vi "Sequencer Main.vi"() -> ()   [LabVIEW 2018] (continued)
              n953 = local read "Barcode"() -> (w1433:string)
              n954 = String Length(string=w1433) -> (length=w1436:i32)
              n955 = Greater?(x=w1436, y=5) -> (0:w1434:bool)
              n956 = case shown="True" w1434 {
                tunnel: w1433 -> [_ w1445]
                tunnel: ["Barcode Err!" w1444] -> w1432
                frame False {
                  n957 = in-place {
                    n958 = global write "Global Variable.vi" "System Status"(T1."Idle" ("System Status")) -> ()
                  }
                  n959 = global write "Global Variable.vi" "Reset BARCODE"(FALSE ("Reset BARCODE")) -> ()
                  n960 = One Button Dialog(message="! - Please Read BARCODE First") -> ()  [unwired: 1 in, 1 out]
                }
                frame True {
                  w1443 = "----------------------------------"
                  w1442 = "\r\n"
                  w1446 = ", "
                  n961 = in-place {
                    n962 = global write "Global Variable.vi" "System Status"(T1."Run Sequencer" ("System Status")) -> ()
                  }
                  n963 = local read "Under Test BOARD"() -> (w1448:string)
                  n964 = local read "Date Time"() -> (w1441:string)
                  n965 = local read "Config"() -> (w1447:string)
                  n966 = global write "Global Variable.vi" "Reset BARCODE"(TRUE ("Reset BARCODE")) -> ()
                  n967 = property on="Run Test" class="Bool"("DisabledEnum"=T18."Disabled and Grayed Out" ("Disabled")) -> ()  [unwired: 2 in, 2 out]
                  n968 = Concatenate Strings(w1448, w1446, w1447, w1446, w1445, w1442, w1443, w1442, w1441, w1442, w1443, w1443, w1442, w1442) -> (w1444:string)
                }
              }
              n969 = local write "LogMsg"(w1432) -> ()
            }
          }
        }
        frame "Run Sequencer" {
          n970 = global read "Sequencer Array.vi" "SEQUENCER Array"() -> (w1452:T16[])
          n971 = Array Size(array=w1452) -> (size(s)=w1457:i32)
          n972 = global write "Global Variable.vi" "Steps Nmb"(w1457) -> ()
          n973 = Greater Than 0?(x=w1457) -> (x > 0?=w1458:bool)
          n974 = case shown="True" w1458 {
            tunnel: w1453 -> [w1461 w1484]
            tunnel: w1456 -> [w1460 w1483]
            tunnel: w1452 -> [_ w1482]
            tunnel: w1453 -> [_ w1475]
            tunnel: w1455 -> [_ w1470]
            tunnel: w1454 -> [_ w1469]
            frame False {
              # "Empty TEST Sequencer"
              n975 = Flush Queue(queue=w1461, error in (no error)=w1460) -> ()  [unwired: 3 out]
              n976 = One Button Dialog(message="Please Load SEQUENCER File") -> ()  [unwired: 1 in, 1 out]
              n977 = global write "Global Variable.vi" "System Status"(T1."Idle" ("System Status")) -> ()
            }
            frame True {
              # "Sys Dig In/Out"
              n978 = Dequeue Element(queue=w1484, error in (no error)=w1483) -> (element=w1466:i32, error out=w1472:errorcluster)  [unwired: 1 in, 2 out]
              n979 = Index Array(array=w1482, index=w1466) -> (element=w1480:T16)
              n980 = global write "Global Variable.vi" "Current Step Nmb"(w1466) -> ()
              n981 = property on="Test Sequencer" class="MCListbox (strict)"("Value"=w1466) -> ()  [unwired: 2 in, 2 out]
              n982 = Unbundle By Name(w1480) -> ("Run/Skip"=w1479:bool, "Step ID"=w1481:u16)
              n983 = flat-sequence {
                tunnel: w1481 -> [w1493]
                tunnel: w1480 -> [w1491]
                tunnel: w1479 -> [w1492]
                tunnel: [w1491] -> w1478
                tunnel: [w1486] -> w1476
                tunnel: w1475 -> [w1486]
                tunnel: w1472 -> [w1485]
                tunnel: [w1490] -> w1473
                tunnel: w1470 -> [w1489]
                tunnel: w1469 -> [w1488]
                tunnel: [w1487] -> w1468
                tunnel: [w1485] -> w1467
                tunnel: w1478 -> [w5997]
                tunnel: [w5996] -> w1477
                tunnel: w1476 -> [w5990]
                tunnel: [w5993] -> w1474
                tunnel: w1473 -> [w5983]
                tunnel: [w5987] -> w1471
                tunnel: w1468 -> [w5991]
                tunnel: w1467 -> [w5992]
                tunnel: [w5983] -> w1465
                tunnel: [w5985] -> w1464
                tunnel: [w5984] -> w1463
                tunnel: w1477 -> [w6131]
                tunnel: w1474 -> [w6124]
                tunnel: w1471 -> [w6129]
                tunnel: w1465 -> [w6128]
                tunnel: w1464 -> [w6123]
                tunnel: w1463 -> [w6130]
                frame #0 {
                  # "Sequencer Array Element"
                  # "Test STEPS Processor"
                  n984 = case shown="True" w1492 {
                    tunnel: w1493 -> [_ w1500]
                    tunnel: w1491 -> [_ w1499]
                    tunnel: [enum16{"Idle", "PASS", "FALSE"}."Idle" ("Step Test Result") w1498] -> w1490
                    tunnel: w1489 -> [_ w1497]
                    tunnel: w1488 -> [_ w1496]
                    tunnel: [_ w1495] -> w1487
                    frame False {
                      # "Step TEST Result"
                    }
                    frame True {
                      # "Run \\ Skip"
                      n985 = case shown="51" w1500 {
                        tunnel: w1499 -> [_ w1505 w1506 w1521 w1647 w1763 w1836 w1998 w2009 w2046 w2131 w2328 w2470 w2603 w2713 w3078 w3442 w3693 w3833 w3925 w4012 w4178 w4330 w4472 w4601 w4710 w5916 w5941]
                        tunnel: [enum16{"Idle", "PASS", "FALSE"}."Idle" ("Step Test Result") enum16{"Idle", "PASS", "FALSE"}."Idle" ("Step Test Result") enum16{"Idle", "PASS", "FALSE"}."Idle" ("Step Test Result") w1509 enum16{"Idle", "PASS", "FALSE"}."Idle" ("Step Test Result") enum16{"Idle", "PASS", "FALSE"}."Idle" ("Step Test Result") w1824 enum16{"Idle", "PASS", "FALSE"}."Idle" ("Step Test Result") enum16{"Idle", "PASS", "FALSE"}."Idle" ("Step Test Result") w2048 w2123 w2327 w2469 w2602 w2710 w3079 w3443 w3694 w3818 w3916 w3991 w4161 w4311 w4466 w4592 w4707 w5907 enum16{"Idle", "PASS", "FALSE"}."PASS" ("Step Test Result")] -> w1498
                        tunnel: w1497 -> [_ _ _ w1515 w1640 w1756 w1829 _ _ _ _ _ _ _ _ _ _ _ _ _ _ _ _ _ _ _ _ w5934]
                        tunnel: w1496 -> [_ _ _ w1514 w1639 w1755 w1828 _ _ _ _ _ _ _ _ _ _ _ _ _ _ _ _ _ _ _ _ w5933]
                        tunnel: [_ _ _ _ _ _ _ _ _ w2045 w2124 w2324 w2466 w2599 w2686 w3071 w3429 w3680 w3817 _ w3990 w4160 w4310 w4465 "SetAWG Gen" ("format string") w4683 w5904 _] -> w1495
                        frame 0, Default {
                          # "Step TEST Result"
                          n986 = One Button Dialog(message="Wrong Step ID!") -> ()  [unwired: 1 in, 1 out]
                        }
                        frame 1 {
                          # "Step TEST Result"
                          # "Label Case"
                          # "Step ID Processing"
                          n987 = Unbundle By Name(w1505) -> ("Step Description"=w1504:string)
                          n988 = local write "Message"(w1504) -> ()
                        }
                        frame 5 {
                          # "Step TEST Result"
                          # "Barcode Case"
                          # "Barcode Operation"
                          n989 = Unbundle By Name(w1506) -> ("Step Description"=w1508:string)
                          n990 = local write "Message"(w1508) -> ()
                        }
                        frame 10 {
                          # "GPIO Case"
                          # "SPI SET Relay"
                          n991 = Unbundle By Name(w1521) -> ("Parameters"=w1520:string, "Step Description"=w1512:string)
                          n992 = global write "Global Variable.vi" "GPIO Mode LUT"(bool[] [FALSE, FALSE, FALSE, FALSE] ("GPIO Mode LUT")) -> ()
                          n993 = call <vilib>:"Acquire Semaphore.vi"("error in (no error)"=w1515, "semaphore"=w1514) -> ("error out"=w1519:errorcluster, "semaphore out"=w1517:T13)  [unwired: 3 in, 1 out]
                          n994 = property on="Msg Str" class="Str"("Value"=w1512) -> ()  [unwired: 2 in, 2 out]
                          n995 = property on="Tab Control Msg" class="TabCtl (strict)"("Value"=T21."Settings" ("Tab Control Msg")) -> (error out=w1513:errorcluster)  [unwired: 2 in, 1 out]
                          n996 = case shown="No Error" w1519 {
                            selector: w1519 -> [w1524 w1634]
                            tunnel: w1520 -> [w1525 _]
                            tunnel: [w1524 w1634] -> w1518
                            tunnel: w1517 -> [w1523 w1633]
                            tunnel: [w1523 w1633] -> w1516
                            tunnel: w1513 -> [_ _]
                            tunnel: [w1522 enum16{"Idle", "PASS", "FALSE"}."Idle" ("Step Test Result")] -> w1509
                            frame No Error {
                              n997 = while {
                                shift-right: [w1530] -> _
                                shift-left: w1525 -> [w1531]
                                tunnel: [w1526] -> w1522
                                stop <- w1529 stop-if-true
                                # "Get Array of Parametrs"
                                n998 = Match Pattern(string=w1531, regular expression=";") -> (before substring=w1527:string, after substring=w1530:string, offset past match=w1528:i32)  [unwired: 1 in, 1 out]
                                n999 = Less Or Equal To 0?(x=w1528) -> (x <= 0?=w1529:bool)
                                n1000 = in-place {
                                in-place-border: w1527 -> [w1567]
                                in-place-border: [w1544] -> w1526
                                # "If True Using\nExtra Settings\n  -nCS <0-4>\n  -ClockRate"
                                # "nCS"
                                # "Addr"
                                n1001 = global read "Global Variable.vi" "GPIO Mode LUT"() -> (w1560:bool[])
                                n1002 = while {
                                shift-right: [w1629] -> _
                                shift-left: w1567 -> [w1630]
                                tunnel: [w1626] -> w1576 mode=indexing
                                stop <- w1628 stop-if-true
                                # "Get Array of Parametrs"
                                n1003 = Match Pattern(string=w1630, regular expression=">") -> (before substring=w1626:string, after substring=w1629:string, offset past match=w1627:i32)  [unwired: 1 in, 1 out]
                                n1004 = Less Than 0?(x=w1627) -> (x < 0?=w1628:bool)
                                }
                                n1005 = Index Array(array=w1576, index #1=0 ("index"), index #2=1 ("index"), index #3=2 ("index")) -> (element #1=w1577:string, element #2=w1578:string, element #3=w1561:string)
                                n1006 = Match Pattern(string=w1561, regular expression="d:") -> (after substring=w1550:string, offset past match=w1566:i32)  [unwired: 1 in, 2 out]
                                n1007 = Match Pattern(string=w1561, regular expression="b:") -> (after substring=w1549:string, offset past match=w1579:i32)  [unwired: 1 in, 2 out]
                                n1008 = Match Pattern(string=w1561, regular expression="s:") -> (after substring=w1547:string, offset past match=w1565:i32)  [unwired: 1 in, 2 out]
                                n1009 = Match Pattern(string=w1561, regular expression="r:") -> (after substring=w1546:string, offset past match=w1562:i32)  [unwired: 1 in, 2 out]
                                n1010 = Greater Than 0?(x=w1566) -> (x > 0?=w1558:bool)
                                n1011 = Greater Than 0?(x=w1562) -> (x > 0?=w1554:bool)
                                n1012 = Greater Than 0?(x=w1579) -> (x > 0?=w1556:bool)
                                n1013 = Greater Than 0?(x=w1565) -> (x > 0?=w1555:bool)
                                n1014 = Replace Array Subset(array=w1560, new element #1=w1558, index #1=0 ("index"), new element #2=w1556, index #2=1 ("index"), new element #3=w1555, index #3=2 ("index"), new element #4=w1554, index #4=3 ("index")) -> (w1548:bool[])
                                n1015 = Boolean Array To Number(Boolean array=w1548) -> (number=w1551:u32)
                                n1016 = case shown="4" w1551 {
                                tunnel: [T24."Set Decimal" ("Mode") T24."Set Decimal" ("Mode") T24."Set Binary" ("Mode") T24."Set Channels" ("Mode") T24."Reset Channels" ("Mode")] -> w1541
                                tunnel: w1550 -> [_ w1610 _ _ _]
                                tunnel: [0 w1609 0 0 0] -> w1536
                                tunnel: [bool[] [FALSE, FALSE, FALSE, FALSE, FALSE, FALSE, FALSE, FALSE, FALSE, FALSE] ("Relays (1-10)") bool[] [FALSE, FALSE, FALSE, FALSE, FALSE, FALSE, FALSE, FALSE, FALSE, FALSE] ("Relays (1-10)") w1614 w1619 w1624] -> w1535
                                tunnel: w1549 -> [_ _ w1612 _ _]
                                tunnel: w1547 -> [_ _ _ w1617 _]
                                tunnel: w1546 -> [_ _ _ _ w1622]
                                frame 0, Default {
                                # "Reset All"
                                n1017 = One Button Dialog(message="Sequencer File Err!") -> ()  [unwired: 1 in, 1 out]
                                }
                                frame 1 {
                                # "Decimale Case"
                                n1018 = Decimal String To Number(string=w1610) -> (number=w1609:i32)  [unwired: 2 in, 1 out]
                                }
                                frame 2 {
                                # "Set Binary Cnannels"
                                n1019 = call "StrBin_To_ArrayBool.vi"("StrBin"=w1612) -> ("Out"=w1615:bool[])  [unwired: 9 in, 1 out]
                                n1020 = Reverse 1D Array(array=w1615) -> (reversed array=w1614:bool[])
                                }
                                frame 4 {
                                # "Set Channels"
                                n1021 = call "StrBin_To_ArrayBool.vi"("StrBin"=w1617) -> ("Out"=w1620:bool[])  [unwired: 9 in, 1 out]
                                n1022 = Reverse 1D Array(array=w1620) -> (reversed array=w1619:bool[])
                                }
                                frame 8 {
                                # "Rest Channels"
                                n1023 = call "StrBin_To_ArrayBool.vi"("StrBin"=w1622) -> ("Out"=w1625:bool[])  [unwired: 9 in, 1 out]
                                n1024 = Reverse 1D Array(array=w1625) -> (reversed array=w1624:bool[])
                                }
                                }
                                n1025 = global write "Global Variable.vi" "GPIO Mode LUT"(w1548) -> ()
                                n1026 = Decimal String To Number(string=w1577) -> (number=w1538:i32)  [unwired: 2 in, 1 out]
                                n1027 = Decimal String To Number(string=w1578) -> (number=w1537:i32)  [unwired: 2 in, 1 out]
                                n1028 = global read "Global Variable.vi" "FTDI SPI Handle"() -> (w1542:u32)
                                n1029 = call "FTDI SPI GPIO Set.vi"("nCS"=w1538, "Relays (1-10)"=w1535, "Mode"=w1541, "Use Extra"=TRUE, "Channel Decimal"=w1536, "Addr"=w1537, "Handler In"=w1542) -> ("error out"=w1543:errorcluster, "LATCH Reg"=w1539:u16, "OK"=w1534:bool)  [unwired: 1 in, 1 out]
                                n1030 = Number To Boolean Array(number=w1539) -> (Boolean array=w1545:bool[])
                                n1031 = global write "Global Variable.vi" "Sys ERR"(w1534) -> ()
                                n1032 = case shown="4" w1537 {
                                tunnel: w1545 -> [_ w1582 w1585 w1588 w1591 w1594 w1597 w1600]
                                frame -1, Default {
                                }
                                frame 0 {
                                n1033 = local read "Switch Relay Modules"() -> (w1584:T5)
                                n1034 = Bundle By Name(cluster=w1584, "SW 0"=w1582) -> (w1583:T5)
                                n1035 = local write "Switch Relay Modules"(w1583) -> ()
                                }
                                frame 1 {
                                n1036 = local read "Switch Relay Modules"() -> (w1587:T5)
                                n1037 = Bundle By Name(cluster=w1587, "SW 1"=w1585) -> (w1586:T5)
                                n1038 = local write "Switch Relay Modules"(w1586) -> ()
                                }
                                frame 2 {
                                n1039 = local read "Switch Relay Modules"() -> (w1590:T5)
                                n1040 = Bundle By Name(cluster=w1590, "SW 2"=w1588) -> (w1589:T5)
                                n1041 = local write "Switch Relay Modules"(w1589) -> ()
                                }
                                frame 3 {
                                n1042 = local read "Switch Relay Modules"() -> (w1593:T5)
                                n1043 = Bundle By Name(cluster=w1593, "SW 3"=w1591) -> (w1592:T5)
                                n1044 = local write "Switch Relay Modules"(w1592) -> ()
                                }
                                frame 4 {
                                n1045 = local read "Switch Relay Modules"() -> (w1596:T5)
                                n1046 = Bundle By Name(cluster=w1596, "SW 4"=w1594) -> (w1595:T5)
                                n1047 = local write "Switch Relay Modules"(w1595) -> ()
                                }
                                frame 5 {
                                n1048 = local read "Switch Relay Modules"() -> (w1599:T5)
                                n1049 = Bundle By Name(cluster=w1599, "SW 5"=w1597) -> (w1598:T5)
                                n1050 = local write "Switch Relay Modules"(w1598) -> ()
                                }
                                frame 6 {
                                n1051 = local read "Switch Relay Modules"() -> (w1602:T5)
                                n1052 = Bundle By Name(cluster=w1602, "SW 6"=w1600) -> (w1601:T5)
                                n1053 = local write "Switch Relay Modules"(w1601) -> ()
                                }
                                }
                                n1054 = global read "Global Variable.vi" "Array Errors"() -> (w1574:errorcluster[])
                                n1055 = case shown="True" w1534 {
                                tunnel: [enum16{"Idle", "PASS", "FALSE"}."Idle" ("Step Test Result") enum16{"Idle", "PASS", "FALSE"}."Idle" ("Step Test Result")] -> w1544
                                frame False {
                                # "Step TEST Result"
                                }
                                frame True {
                                # "Step TEST Result"
                                }
                                }
                                n1056 = Replace Array Subset(array=w1574, new element=w1543, index=10) -> (w1575:errorcluster[])
                                n1057 = global write "Global Variable.vi" "Array Errors"(w1575) -> ()
                                n1058 = Wait (ms)(milliseconds to wait=u32 50) -> ()  [unwired: 1 out]
                                }
                              }
                            }
                            frame Error {
                              # "Step TEST Result"
                            }
                          }
                          n1059 = call <vilib>:"Release Semaphore.vi"("error in (no error)"=w1518, "semaphore"=w1516) -> ()  [unwired: 4 in, 2 out]
                        }
                        frame 11 {
                          # "GPIO SYS Case"
                          # "Step TEST Result"
                          # "SPI SET DIGOUT SYS"
                          n1060 = Unbundle By Name(w1647) -> ("Parameters"=w1645:string, "Step Description"=w1637:string)
                          n1061 = global write "Global Variable.vi" "GPIO Mode LUT"(bool[] [FALSE, FALSE, FALSE, FALSE] ("GPIO Mode LUT")) -> ()
                          n1062 = property on="Tab Control Msg" class="TabCtl (strict)"("Value"=T21."Msg" ("Tab Control Msg")) -> (error out=w1638:errorcluster)  [unwired: 2 in, 1 out]
                          n1063 = call <vilib>:"Acquire Semaphore.vi"("error in (no error)"=w1640, "semaphore"=w1639) -> ("error out"=w1644:errorcluster, "semaphore out"=w1642:T13)  [unwired: 3 in, 1 out]
                          n1064 = property on="Msg Str" class="Str"("Value"=w1637) -> ()  [unwired: 2 in, 2 out]
                          n1065 = case shown="No Error" w1644 {
                            selector: w1644 -> [w1649 w1750]
                            tunnel: w1645 -> [w1650 _]
                            tunnel: [w1649 w1750] -> w1643
                            tunnel: w1642 -> [w1648 w1749]
                            tunnel: [w1648 w1749] -> w1641
                            tunnel: w1638 -> [_ _]
                            frame No Error {
                              n1066 = while {
                                shift-right: [w1654] -> _
                                shift-left: w1650 -> [w1655]
                                stop <- w1653 stop-if-true
                                # "Get Array of Parametrs"
                                n1067 = Match Pattern(string=w1655, regular expression=";") -> (before substring=w1651:string, after substring=w1654:string, offset past match=w1652:i32)  [unwired: 1 in, 1 out]
                                n1068 = Less Or Equal To 0?(x=w1652) -> (x <= 0?=w1653:bool)
                                n1069 = in-place {
                                in-place-border: w1651 -> [w1686]
                                # "If True Using\nExtra Settings\n  -nCS <0-4>\n  -ClockRate"
                                # "nCS"
                                # "Addr"
                                n1070 = global read "Global Variable.vi" "GPIO Mode LUT"() -> (w1679:bool[])
                                n1071 = while {
                                shift-right: [w1746] -> _
                                shift-left: w1686 -> [w1747]
                                tunnel: [w1743] -> w1695 mode=indexing
                                stop <- w1745 stop-if-true
                                # "Get Array of Parametrs"
                                n1072 = Match Pattern(string=w1747, regular expression=">") -> (before substring=w1743:string, after substring=w1746:string, offset past match=w1744:i32)  [unwired: 1 in, 1 out]
                                n1073 = Less Than 0?(x=w1744) -> (x < 0?=w1745:bool)
                                }
                                n1074 = Index Array(array=w1695, index #1=0 ("index"), index #2=1 ("index"), index #3=2 ("index")) -> (element #1=w1696:string, element #2=w1697:string, element #3=w1680:string)
                                n1075 = Match Pattern(string=w1680, regular expression="d:") -> (after substring=w1669:string, offset past match=w1685:i32)  [unwired: 1 in, 2 out]
                                n1076 = Match Pattern(string=w1680, regular expression="b:") -> (after substring=w1668:string, offset past match=w1698:i32)  [unwired: 1 in, 2 out]
                                n1077 = Match Pattern(string=w1680, regular expression="s:") -> (after substring=w1666:string, offset past match=w1684:i32)  [unwired: 1 in, 2 out]
                                n1078 = Match Pattern(string=w1680, regular expression="r:") -> (after substring=w1665:string, offset past match=w1681:i32)  [unwired: 1 in, 2 out]
                                n1079 = Greater Than 0?(x=w1685) -> (x > 0?=w1677:bool)
                                n1080 = Greater Than 0?(x=w1681) -> (x > 0?=w1673:bool)
                                n1081 = Greater Than 0?(x=w1698) -> (x > 0?=w1675:bool)
                                n1082 = Greater Than 0?(x=w1684) -> (x > 0?=w1674:bool)
                                n1083 = Replace Array Subset(array=w1679, new element #1=w1677, index #1=0 ("index"), new element #2=w1675, index #2=1 ("index"), new element #3=w1674, index #3=2 ("index"), new element #4=w1673, index #4=3 ("index")) -> (w1667:bool[])
                                n1084 = Boolean Array To Number(Boolean array=w1667) -> (number=w1670:u32)
                                n1085 = case shown="0, Default" w1670 {
                                tunnel: [T23."Set Decimal" ("Mode") T23."Set Decimal" ("Mode") T23."Set Binary" ("Mode") T23."Set Channels" ("Mode") T23."Reset Channels" ("Mode")] -> _
                                tunnel: w1669 -> [_ w1726 _ _ _]
                                tunnel: [0 w1725 0 0 0] -> _
                                tunnel: [bool[] [FALSE, FALSE, FALSE, FALSE, FALSE, FALSE, FALSE, FALSE, FALSE, FALSE] ("Relays (1-10)") bool[] [FALSE, FALSE, FALSE, FALSE, FALSE, FALSE, FALSE, FALSE, FALSE, FALSE] ("Relays (1-10)") w1730 w1735 w1741] -> w1657
                                tunnel: w1668 -> [_ _ w1728 _ _]
                                tunnel: w1666 -> [_ _ _ w1733 _]
                                tunnel: w1665 -> [_ _ _ _ w1739]
                                frame 0, Default {
                                n1086 = One Button Dialog(message="Sequencer File Err!") -> ()  [unwired: 1 in, 1 out]
                                }
                                frame 1 {
                                # "Decimale Case"
                                n1087 = Decimal String To Number(string=w1726) -> (number=w1725:i32)  [unwired: 2 in, 1 out]
                                }
                                frame 2 {
                                # "Set Binary Cnannels"
                                n1088 = call "StrBin_To_ArrayBool.vi"("StrBin"=w1728) -> ("Out"=w1732:bool[])  [unwired: 9 in, 1 out]
                                n1089 = Reverse 1D Array(array=w1732) -> (reversed array=w1730:bool[])
                                }
                                frame 4 {
                                # "Set Channels"
                                n1090 = call "StrBin_To_ArrayBool.vi"("StrBin"=w1733) -> ("Out"=w1737:bool[])  [unwired: 9 in, 1 out]
                                n1091 = Reverse 1D Array(array=w1737) -> (reversed array=w1735:bool[])
                                }
                                frame 8 {
                                # "Rest Channels"
                                n1092 = call "StrBin_To_ArrayBool.vi"("StrBin"=w1739) -> ("Out"=w1742:bool[])  [unwired: 9 in, 1 out]
                                n1093 = Reverse 1D Array(array=w1742) -> (reversed array=w1741:bool[])
                                }
                                }
                                n1094 = global write "Global Variable.vi" "GPIO Mode LUT"(w1667) -> ()
                                n1095 = Decimal String To Number(string=w1696) -> (number=w1659:i32)  [unwired: 2 in, 1 out]
                                n1096 = Decimal String To Number(string=w1697) -> (number=w1661:i32)  [unwired: 2 in, 1 out]
                                n1097 = global read "Global Variable.vi" "FTDI SPI Handle"() -> (w1660:u32)
                                n1098 = call "FTDI SPI SYS Set.vi"("nCS"=w1659, "Set Out (0-7)"=w1657, "Use Extra"=TRUE, "Addr"=w1661, "Handler In"=w1660) -> ("error out"=w1662:errorcluster, "Latch Reg"=w1658:u32)  [unwired: 4 in, 1 out]
                                n1099 = Number To Boolean Array(number=w1658) -> (Boolean array=w1664:bool[])
                                n1100 = case shown="6" w1661 {
                                tunnel: w1664 -> [_ w1699 w1702 w1705 w1708 w1711 w1714 w1717]
                                frame -1, Default {
                                }
                                frame 0 {
                                n1101 = local read "Switch Relay Modules"() -> (w1701:T5)
                                n1102 = Bundle By Name(cluster=w1701, "SW 0"=w1699) -> (w1700:T5)
                                n1103 = local write "Switch Relay Modules"(w1700) -> ()
                                }
                                frame 1 {
                                n1104 = local read "Switch Relay Modules"() -> (w1704:T5)
                                n1105 = Bundle By Name(cluster=w1704, "SW 1"=w1702) -> (w1703:T5)
                                n1106 = local write "Switch Relay Modules"(w1703) -> ()
                                }
                                frame 2 {
                                n1107 = local read "Switch Relay Modules"() -> (w1707:T5)
                                n1108 = Bundle By Name(cluster=w1707, "SW 2"=w1705) -> (w1706:T5)
                                n1109 = local write "Switch Relay Modules"(w1706) -> ()
                                }
                                frame 3 {
                                n1110 = local read "Switch Relay Modules"() -> (w1710:T5)
                                n1111 = Bundle By Name(cluster=w1710, "SW 3"=w1708) -> (w1709:T5)
                                n1112 = local write "Switch Relay Modules"(w1709) -> ()
                                }
                                frame 4 {
                                n1113 = local read "Switch Relay Modules"() -> (w1713:T5)
                                n1114 = Bundle By Name(cluster=w1713, "SW 4"=w1711) -> (w1712:T5)
                                n1115 = local write "Switch Relay Modules"(w1712) -> ()
                                }
                                frame 5 {
                                n1116 = local read "Switch Relay Modules"() -> (w1716:T5)
                                n1117 = Bundle By Name(cluster=w1716, "SW 5"=w1714) -> (w1715:T5)
                                n1118 = local write "Switch Relay Modules"(w1715) -> ()
                                }
                                frame 6 {
                                n1119 = local read "Switch Relay Modules"() -> (w1719:T5)
                                n1120 = Bundle By Name(cluster=w1719, "SW 6"=w1717) -> (w1718:T5)
                                n1121 = local write "Switch Relay Modules"(w1718) -> ()
                                }
                                }
                                n1122 = global read "Global Variable.vi" "Array Errors"() -> (w1693:errorcluster[])
                                n1123 = Replace Array Subset(array=w1693, new element=w1662, index=10) -> (w1694:errorcluster[])
                                n1124 = global write "Global Variable.vi" "Array Errors"(w1694) -> ()
                                }
                              }
                            }
                            frame Error {
                            }
                          }
                          n1125 = call <vilib>:"Release Semaphore.vi"("error in (no error)"=w1643, "semaphore"=w1641) -> ()  [unwired: 4 in, 2 out]
                        }
                        frame 14 {
                          # "GPIO BASE DigOut Case"
                          # "Step TEST Result"
                          # "SPI SET BASE DigOut"
                          n1126 = Unbundle By Name(w1763) -> ("Parameters"=w1761:string, "Step Description"=w1753:string)
                          n1127 = global write "Global Variable.vi" "GPIO Mode LUT"(bool[] [FALSE, FALSE, FALSE, FALSE] ("GPIO Mode LUT")) -> ()
                          n1128 = call <vilib>:"Acquire Semaphore.vi"("error in (no error)"=w1756, "semaphore"=w1755) -> ("error out"=w1760:errorcluster, "semaphore out"=w1758:T13)  [unwired: 3 in, 1 out]
                          n1129 = property on="Msg Str" class="Str"("Value"=w1753) -> ()  [unwired: 2 in, 2 out]
                          n1130 = property on="Tab Control Msg" class="TabCtl (strict)"("Value"=T21."Msg" ("Tab Control Msg")) -> (error out=w1754:errorcluster)  [unwired: 2 in, 1 out]
                          n1131 = case shown="No Error" w1760 {
                            selector: w1760 -> [w1765 w1822]
                            tunnel: w1761 -> [w1766 _]
                            tunnel: [w1765 w1822] -> w1759
                            tunnel: w1758 -> [w1764 w1821]
                            tunnel: [w1764 w1821] -> w1757
                            tunnel: w1754 -> [_ _]
                            frame No Error {
                              n1132 = while {
                                shift-right: [w1770] -> _
                                shift-left: w1766 -> [w1771]
                                stop <- w1769 stop-if-true
                                # "Get Array of Parametrs"
                                n1133 = Match Pattern(string=w1771, regular expression=";") -> (before substring=w1767:string, after substring=w1770:string, offset past match=w1768:i32)  [unwired: 1 in, 1 out]
                                n1134 = Less Or Equal To 0?(x=w1768) -> (x <= 0?=w1769:bool)
                                n1135 = in-place {
                                in-place-border: w1767 -> [w1794]
                                w1790 = 2 ("length (rest)")
                                # "If True Using\nExtra Settings\n  -nCS <0-4>\n  -ClockRate"
                                # "nCS"
                                # "Addr"
                                n1136 = while {
                                shift-right: [w1818] -> _
                                shift-left: w1794 -> [w1819]
                                tunnel: [w1815] -> w1801 mode=indexing
                                stop <- w1817 stop-if-true
                                # "Get Array of Parametrs"
                                n1137 = Match Pattern(string=w1819, regular expression=">") -> (before substring=w1815:string, after substring=w1818:string, offset past match=w1816:i32)  [unwired: 1 in, 1 out]
                                n1138 = Less Than 0?(x=w1816) -> (x < 0?=w1817:bool)
                                }
                                n1139 = Index Array(array=w1801, index #1=0 ("index"), index #2=1 ("index"), index #3=2 ("index")) -> (element #1=w1802:string, element #2=w1803:string, element #3=w1791:string)
                                n1140 = String Subset(string=w1791, offset (0)=w1790, length (rest)=8 ("length (rest)")) -> (substring=w1781:string)
                                n1141 = String Subset(string=w1791, offset (0)=0, length (rest)=w1790) -> (substring=w1792:string)
                                n1142 = call "StrBin_To_ArrayBool_8Bit.vi"("StrBin"=w1781) -> ("Out"=w1780:bool[])  [unwired: 9 in, 1 out]
                                n1143 = Reverse 1D Array(array=w1780) -> (reversed array=w1773:bool[])
                                n1144 = case shown="\"Idle\", Default" w1792 {
                                tunnel: [w1806 w1808 bool[] [FALSE, FALSE, FALSE, FALSE, FALSE, FALSE, FALSE, FALSE]] -> w1785
                                tunnel: [w1806 bool[] [FALSE, FALSE, FALSE, FALSE, FALSE, FALSE, FALSE, FALSE] w1812] -> w1775
                                tunnel: [w1806 w1808 w1812] -> _
                                tunnel: [w1805 w1809 w1813] -> w1782
                                tunnel: w1773 -> [_ w1808 w1812]
                                tunnel: [0 0 1] -> w1774
                                frame "Idle", Default {
                                w1805 = u16 0 items=["Ch-A", "Ch-B"] ("Set Channel")
                                w1806 = bool[] [FALSE, FALSE, FALSE, FALSE, FALSE, FALSE, FALSE, FALSE]
                                }
                                frame "A:" {
                                w1809 = u16 0 items=["Ch-A", "Ch-B"] ("Set Channel")
                                }
                                frame "B:" {
                                w1813 = u16 1 items=["Ch-A", "Ch-B"] ("Set Channel")
                                }
                                }
                                n1145 = Decimal String To Number(string=w1802) -> (number=w1783:i32)  [unwired: 2 in, 1 out]
                                n1146 = Decimal String To Number(string=w1803) -> (number=w1786:i32)  [unwired: 2 in, 1 out]
                                n1147 = global read "Global Variable.vi" "FTDI SPI Handle"() -> (w1788:u32)
                                n1148 = call "FTDI SPI BASE AB-Set.vi"("nCS"=w1783, "Set Out-B (0-7)"=w1775, "Set Out-A (0-7)"=w1785, "Use Extra"=TRUE, "Set Channel"=w1782, "Addr"=w1786, "Handler In"=w1788) -> ("error out"=w1784:errorcluster)  [unwired: 2 in, 2 out]
                                n1149 = global read "Global Variable.vi" "Array Errors"() -> (w1799:errorcluster[])
                                n1150 = Replace Array Subset(array=bool[][] [] ("BASE"), new element=w1773, index (row)=w1774) -> (w1776:bool[][])  [unwired: 1 in]
                                n1151 = local read "Switch Relay Modules"() -> (w1779:T5)
                                n1152 = Replace Array Subset(array=w1799, new element=w1784, index=10) -> (w1800:errorcluster[])
                                n1153 = Bundle By Name(cluster=w1779, "BASE"=w1776) -> (w1778:T5)
                                n1154 = local write "Switch Relay Modules"(w1778) -> ()
                                n1155 = global write "Global Variable.vi" "Array Errors"(w1800) -> ()
                                }
                              }
                            }
                            frame Error {
                            }
                          }
                          n1156 = call <vilib>:"Release Semaphore.vi"("error in (no error)"=w1759, "semaphore"=w1757) -> ()  [unwired: 4 in, 2 out]
                        }
                        frame 12 {
                          # "Reset Modules Case"
                          # "Reset Modules"
                          n1157 = Unbundle By Name(w1836) -> ("Parameters"=w1834:string, "Step Description"=w1826:string)
                          n1158 = property on="Tab Control Msg" class="TabCtl (strict)"("Value"=T21."Settings" ("Tab Control Msg")) -> (error out=w1827:errorcluster)  [unwired: 2 in, 1 out]
                          n1159 = call <vilib>:"Acquire Semaphore.vi"("error in (no error)"=w1829, "semaphore"=w1828) -> ("error out"=w1833:errorcluster, "semaphore out"=w1831:T13)  [unwired: 3 in, 1 out]
                          n1160 = property on="Msg Str" class="Str"("Value"=w1826) -> ()  [unwired: 2 in, 2 out]
                          n1161 = case shown="No Error" w1833 {
                            selector: w1833 -> [w1841 w1990]
                            tunnel: w1834 -> [w1842 _]
                            tunnel: [w1841 w1990] -> w1832
                            tunnel: w1831 -> [w1840 w1989]
                            tunnel: [w1840 w1989] -> w1830
                            tunnel: w1827 -> [_ _]
                            tunnel: [w1839 FALSE ("OK")] -> w1823
                            frame No Error {
                              n1162 = while {
                                shift-right: [w1847] -> _
                                shift-left: w1842 -> [w1848]
                                tunnel: [w1843] -> w1839
                                stop <- w1846 stop-if-true
                                # "Get Array of Parametrs"
                                n1163 = Match Pattern(string=w1848, regular expression=";") -> (before substring=w1844:string, after substring=w1847:string, offset past match=w1845:i32)  [unwired: 1 in, 1 out]
                                n1164 = Less Or Equal To 0?(x=w1845) -> (x <= 0?=w1846:bool)
                                n1165 = in-place {
                                in-place-border: w1844 -> [w1873]
                                in-place-border: [w1858] -> w1843
                                n1166 = flat-sequence {
                                tunnel: w1873 -> [w1896]
                                tunnel: [w1887] -> w1872
                                tunnel: [w1886] -> w1871
                                tunnel: [w1878] -> w1868
                                tunnel: [w1877] -> w1866
                                tunnel: [w1876] -> w1865
                                tunnel: [w1884] -> w1863
                                tunnel: [w1881] -> w1854
                                tunnel: [w1876] -> w1853
                                tunnel: [w1875] -> w1851
                                tunnel: w1872 -> [w1923]
                                tunnel: w1871 -> [w1922]
                                tunnel: [w1922] -> w1870
                                tunnel: [w1921] -> w1869
                                tunnel: w1868 -> [w1921]
                                tunnel: [w1920] -> w1867
                                tunnel: w1866 -> [w1920]
                                tunnel: w1865 -> [w1919]
                                tunnel: [w1919] -> w1864
                                tunnel: w1863 -> [w1918]
                                tunnel: [w1917] -> w1860
                                tunnel: [w1916] -> w1857
                                tunnel: [w1915] -> w1855
                                tunnel: w1854 -> [w1915]
                                tunnel: w1853 -> [w1917]
                                tunnel: w1851 -> [w1916]
                                tunnel: w1870 -> [w1956]
                                tunnel: w1869 -> [w1948]
                                tunnel: w1867 -> [w1947]
                                tunnel: w1864 -> [_]
                                tunnel: [w1956] -> w1862
                                tunnel: [w1946] -> w1861
                                tunnel: w1860 -> [w1946]
                                tunnel: [w1955] -> w1859
                                tunnel: w1857 -> [w1954]
                                tunnel: [w1954] -> w1856
                                tunnel: w1855 -> [w1949]
                                tunnel: [w1952] -> w1852
                                tunnel: [w1945] -> w1850
                                tunnel: w1862 -> [w1966]
                                tunnel: w1861 -> [w1965]
                                tunnel: w1859 -> [w1964]
                                tunnel: [w1960] -> w1858
                                tunnel: w1856 -> [w1957]
                                tunnel: w1852 -> [w1959]
                                tunnel: w1850 -> [w1960]
                                frame #0 {
                                # "Delay(Passive)"
                                # "Delay (Active)"
                                # "nCS"
                                # "Addr"
                                n1167 = while {
                                shift-right: [w1912] -> _
                                shift-left: w1896 -> [w1913]
                                tunnel: [w1909] -> w1900 mode=indexing
                                stop <- w1911 stop-if-true
                                # "Get Array of Parametrs"
                                n1168 = Match Pattern(string=w1913, regular expression=">") -> (before substring=w1909:string, after substring=w1912:string, offset past match=w1910:i32)  [unwired: 1 in, 1 out]
                                n1169 = Less Than 0?(x=w1910) -> (x < 0?=w1911:bool)
                                }
                                n1170 = case shown="0, Default" 0 {
                                tunnel: [0 4 2 6 1 5 3 7] -> _
                                frame 0, Default {
                                }
                                frame 1 {
                                }
                                frame 2 {
                                }
                                frame 3 {
                                }
                                frame 4 {
                                }
                                frame 5 {
                                }
                                frame 6 {
                                }
                                frame 7 {
                                }
                                }
                                n1171 = Index Array(array=w1900, index #1=0 ("index"), index #2=1 ("index"), index #3=2 ("index")) -> (element #1=w1895:string, element #2=w1894:string, element #3=w1892:string, element #4=w1889:string, element #5=w1888:string)  [unwired: 2 in]
                                n1172 = To Lower Case(string=w1892) -> (all lower case string=w1891:string)
                                n1173 = Match Pattern(string=w1891, regular expression="rst:") -> (after substring=w1890:string)  [unwired: 1 in, 3 out]
                                n1174 = global read "Global Variable.vi" "FTDI SPI Handle"() -> (w1880:u32)
                                n1175 = Decimal String To Number(string=w1889) -> (number=w1887:i32)  [unwired: 2 in, 1 out]
                                n1176 = Decimal String To Number(string=w1895) -> (number=w1878:i32)  [unwired: 2 in, 1 out]
                                n1177 = Decimal String To Number(string=w1894) -> (number=w1876:i32)  [unwired: 2 in, 1 out]
                                n1178 = call "StrBin_To_ArrayBool.vi"("StrBin"=w1890) -> ("Out"=w1885:bool[])  [unwired: 9 in, 1 out]
                                n1179 = Reverse 1D Array(array=w1885) -> (reversed array=w1877:bool[])
                                n1180 = Decimal String To Number(string=w1888) -> (number=w1886:i32)  [unwired: 2 in, 1 out]
                                n1181 = call "FTDI SPI GPIO Set.vi"("nCS"=w1878, "Relays (1-10)"=w1877, "Mode"=T23."Set Channels", "Use Extra"=TRUE, "Addr"=w1876, "Handler In"=w1880) -> ("error out"=w1875:errorcluster, "LATCH Reg"=w1874:u16, "Handler Out"=w1881:u32)  [unwired: 2 in, 1 out]
                                n1182 = Number To Boolean Array(number=w1874) -> (Boolean array=w1884:bool[])
                                }
                                frame #1 {
                                n1183 = case shown="2" w1917 {
                                tunnel: w1918 -> [_ w1924 w1927 w1930 w1933 w1936 w1939 w1942]
                                frame -1, Default {
                                }
                                frame 0 {
                                n1184 = local read "Switch Relay Modules"() -> (w1926:T5)
                                n1185 = Bundle By Name(cluster=w1926, "SW 0"=w1924) -> (w1925:T5)
                                n1186 = local write "Switch Relay Modules"(w1925) -> ()
                                }
                                frame 1 {
                                n1187 = local read "Switch Relay Modules"() -> (w1929:T5)
                                n1188 = Bundle By Name(cluster=w1929, "SW 1"=w1927) -> (w1928:T5)
                                n1189 = local write "Switch Relay Modules"(w1928) -> ()
                                }
                                frame 2 {
                                n1190 = local read "Switch Relay Modules"() -> (w1932:T5)
                                n1191 = Bundle By Name(cluster=w1932, "SW 2"=w1930) -> (w1931:T5)
                                n1192 = local write "Switch Relay Modules"(w1931) -> ()
                                }
                                frame 3 {
                                n1193 = local read "Switch Relay Modules"() -> (w1935:T5)
                                n1194 = Bundle By Name(cluster=w1935, "SW 3"=w1933) -> (w1934:T5)
                                n1195 = local write "Switch Relay Modules"(w1934) -> ()
                                }
                                frame 4 {
                                n1196 = local read "Switch Relay Modules"() -> (w1938:T5)
                                n1197 = Bundle By Name(cluster=w1938, "SW 4"=w1936) -> (w1937:T5)
                                n1198 = local write "Switch Relay Modules"(w1937) -> ()
                                }
                                frame 5 {
                                n1199 = local read "Switch Relay Modules"() -> (w1941:T5)
                                n1200 = Bundle By Name(cluster=w1941, "SW 5"=w1939) -> (w1940:T5)
                                n1201 = local write "Switch Relay Modules"(w1940) -> ()
                                }
                                frame 6 {
                                n1202 = local read "Switch Relay Modules"() -> (w1944:T5)
                                n1203 = Bundle By Name(cluster=w1944, "SW 6"=w1942) -> (w1943:T5)
                                n1204 = local write "Switch Relay Modules"(w1943) -> ()
                                }
                                }
                                n1205 = Wait (ms)(milliseconds to wait=w1923) -> ()  [unwired: 1 out]
                                }
                                frame #2 {
                                # "Addr"
                                # "nCS"
                                n1206 = call "FTDI SPI GPIO Set.vi"("nCS"=w1948, "Relays (1-10)"=w1947, "Mode"=T23."Reset Channels", "Use Extra"=TRUE, "Addr"=w1946, "Handler In"=w1949) -> ("error out"=w1952:errorcluster, "LATCH Reg"=w1951:u16, "OK"=w1945:bool)  [unwired: 2 in, 1 out]
                                n1207 = Number To Boolean Array(number=w1951) -> (Boolean array=w1955:bool[])
                                }
                                frame #3 {
                                n1208 = global read "Global Variable.vi" "Array Errors"() -> (w1962:errorcluster[])
                                n1209 = case shown="2" w1965 {
                                tunnel: w1964 -> [_ w1967 w1970 w1973 w1976 w1979 w1982 w1985]
                                frame -1, Default {
                                }
                                frame 0 {
                                n1210 = local read "Switch Relay Modules"() -> (w1969:T5)
                                n1211 = Bundle By Name(cluster=w1969, "SW 0"=w1967) -> (w1968:T5)
                                n1212 = local write "Switch Relay Modules"(w1968) -> ()
                                }
                                frame 1 {
                                n1213 = local read "Switch Relay Modules"() -> (w1972:T5)
                                n1214 = Bundle By Name(cluster=w1972, "SW 1"=w1970) -> (w1971:T5)
                                n1215 = local write "Switch Relay Modules"(w1971) -> ()
                                }
                                frame 2 {
                                n1216 = local read "Switch Relay Modules"() -> (w1975:T5)
                                n1217 = Bundle By Name(cluster=w1975, "SW 2"=w1973) -> (w1974:T5)
                                n1218 = local write "Switch Relay Modules"(w1974) -> ()
                                }
                                frame 3 {
                                n1219 = local read "Switch Relay Modules"() -> (w1978:T5)
                                n1220 = Bundle By Name(cluster=w1978, "SW 3"=w1976) -> (w1977:T5)
                                n1221 = local write "Switch Relay Modules"(w1977) -> ()
                                }
                                frame 4 {
                                n1222 = local read "Switch Relay Modules"() -> (w1981:T5)
                                n1223 = Bundle By Name(cluster=w1981, "SW 4"=w1979) -> (w1980:T5)
                                n1224 = local write "Switch Relay Modules"(w1980) -> ()
                                }
                                frame 5 {
                                n1225 = local read "Switch Relay Modules"() -> (w1984:T5)
                                n1226 = Bundle By Name(cluster=w1984, "SW 5"=w1982) -> (w1983:T5)
                                n1227 = local write "Switch Relay Modules"(w1983) -> ()
                                }
                                frame 6 {
                                n1228 = local read "Switch Relay Modules"() -> (w1987:T5)
                                n1229 = Bundle By Name(cluster=w1987, "SW 6"=w1985) -> (w1986:T5)
                                n1230 = local write "Switch Relay Modules"(w1986) -> ()
                                }
                                }
                                n1231 = Merge Errors(w1959, w1957) -> (w1958:errorcluster)
                                n1232 = Wait (ms)(milliseconds to wait=w1966) -> ()  [unwired: 1 out]
                                n1233 = Replace Array Subset(array=w1962, new element=w1958, index=10) -> (w1963:errorcluster[])
                                n1234 = global write "Global Variable.vi" "Array Errors"(w1963) -> ()
                                }
                                }
                                }
                              }
                            }
                            frame Error {
                            }
                          }
                          n1235 = case shown="False" w1823 {
                            tunnel: [enum16{"Idle", "PASS", "FALSE"}."FALSE" ("Step Test Result") enum16{"Idle", "PASS", "FALSE"}."Idle" ("Step Test Result")] -> w1824
                            frame False {
                              # "Step TEST Result"
                            }
                            frame True {
                              # "Step TEST Result"
                            }
                          }
                          n1236 = case shown="True" FALSE {
                            frame False {
                            }
                            frame True {
                              n1237 = Wait (ms)(milliseconds to wait=u32 250) -> ()  [unwired: 1 out]
                            }
                          }
                          n1238 = call <vilib>:"Release Semaphore.vi"("error in (no error)"=w1832, "semaphore"=w1830) -> ()  [unwired: 4 in, 2 out]
                        }
                        frame 13 {
                          # "Sys Delay Case"
                          # "Step TEST Result"
                          # "System Delay"
                          n1239 = Unbundle By Name(w1998) -> ("Parameters"=w1994:string, "Step Description"=w1996:string)
                          n1240 = property on="Tab Control Msg" class="TabCtl (strict)"("Value"=T21."Msg" ("Tab Control Msg")) -> (error out=w1993:errorcluster)  [unwired: 2 in, 1 out]
                          n1241 = property on="Msg Str" class="Str"(error in=w1993, "Value"=w1996) -> (error out=w1992:errorcluster)  [unwired: 1 in, 1 out]
                          n1242 = in-place {
                            in-place-border: w1994 -> [w1999]
                            in-place-border: w1992 -> [_]
                            n1243 = Decimal String To Number(string=w1999) -> (number=w2001:i32)  [unwired: 2 in, 1 out]
                            n1244 = Greater Than 0?(x=w2001) -> (x > 0?=w2000:bool)
                            n1245 = case shown="True" w2000 {
                              tunnel: w2001 -> [_ w2002]
                              frame False {
                              }
                              frame True {
                                n1246 = Wait (ms)(milliseconds to wait=w2002) -> ()  [unwired: 1 out]
                              }
                            }
                          }
                        }
                        frame 15 {
                          # "PS Set Case"
                          # "Step TEST Result"
                          # "Power Supplay Set"
